vi "Calibration curve generator (for plot visualisation).vi"(0 "Calibration data":T1={"X cal.[]"=[0.18323830295620053, 0.5022759108677167, 0.5926494582411277, 0.6661572393359195, 0.7738522670991032, 0.8056162976693839, 0.8978854253288069, 0.9131465104685323, 0.998198602505461, 1.0026536354542668, 1.0697031684682123, 1.0921294784978217, 1.12634848007751], "Re cal.[]"=[0.05836901900647489, 0.22234941748039563, 0.3015014894413766, 0.37907259878050203, 0.5315212662031547, 0.5843186336351215, 0.7493379557739939, 0.7811312845686427, 0.9579100635301298, 0.968544779466997, 1.1278235480081842, 1.1845542549316277, 1.2707750850078616], "a1[]"=[0.5139845410306613, 0.694908421100499, 0.9655549133380104, 1.2354182702612118, 1.5388668488196042, 1.7253155968767342, 1.935875310920986, 2.080885331144939, 2.2328002605238204, 2.3813313947618693, 2.452594226248764, 2.5246632991683033], "a2[]"=[-0.567092642319511, 3.0111150428522957, -0.009461861177446703, 2.2004140825264833, 5.776179850523374, -0.22907956125341525, 19.477407826803766, -1.871103511573675, 70.58084557623488, -1.3220160025433672, 7.094218596447346, -0.2914365144530001], "a3[]"=[1.7775103256064757, -11.166529475918521, 16.733581628717324, -4.900141213800908, -59.63298736273686, 9.899216022714324, -643.3109334585097, 21.66651332028892, -8067.401298929666, 18.428518110921583, -163.1245085960374, 4.25840177969994]}, 5 "Overheat ratio":dbl=1.7, 7 "Gain":dbl=10.0, 9 "Offset (V)":dbl=0.512, 11 "N pts":i32=200, 12 "Vout_start (V)":dbl=0.0915928 format="%0.2f", 13 "Vout_end (V)":dbl=2.56055 format="%0.2f", 14 "Ta (°C)":dbl=20.43) -> ()   [LabVIEW 2022 SP3]
doc: "Generate spline interpolated calibration curve for plotting or testing purposes.\nPN 19-FEB-24."
uses:
  Ctls/Calibration data.ctl
  <vilib>/Analysis/1siggen.llb/Ramp Pattern by Samples.vi
  <vilib>/Analysis/NI_AALBase.lvlib
panel:
  out "U against Vout":cluster{dbl[], dbl[]}(graph)={[0.0915928, 0.10399962010050251, 0.11640644020100503, 0.12881326030150753, 0.14122008040201006, 0.15362690050251257, 0.16603372060301508, 0.1784405407035176, 0.1908473608040201, 0.20325418090452263, 0.21566100100502514, 0.22806782110552765, 0.24047464120603015, 0.25288146130653266, 0.2652882814070352, 0.27769510150753773, 0.2901019216080402, 0.3025087417085427, 0.31491556180904523, 0.32732238190954777, 0.3397292020100503, 0.3521360221105527, 0.36454284221105526, 0.3769496623115578, 0.38935648241206033, 0.40176330251256287, 0.4141701226130653, 0.42657694271356783, 0.43898376281407037, 0.4513905829145729, 0.46379740301507544, 0.47620422311557786, 0.4886110432160804, 0.5010178633165829, 0.5134246834170855, 0.525831503517588, 0.5382383236180904, 0.550645143718593, 0.5630519638190955, 0.575458783919598, 0.5878656040201006, 0.6002724241206031, 0.6126792442211055, 0.6250860643216081, 0.6374928844221106, 0.6498997045226131, 0.6623065246231157, 0.6747133447236181, 0.6871201648241206, 0.6995269849246232, 0.7119338050251257, 0.7243406251256282, 0.7367474452261307, 0.7491542653266332, 0.7615610854271357, 0.7739679055276383, 0.7863747256281408, 0.7987815457286432, 0.8111883658291458, 0.8235951859296483, 0.8360020060301508, 0.8484088261306534, 0.8608156462311558, 0.8732224663316583, 0.8856292864321609, 0.8980361065326634, 0.910442926633166, 0.9228497467336684, 0.9352565668341709, 0.9476633869346734, 0.960070207035176, 0.9724770271356785, 0.9848838472361809, 0.9972906673366835, 1.009697487437186, 1.0221043075376886, 1.034511127638191, 1.0469179477386934, 1.059324767839196, 1.0717315879396985, 1.084138408040201, 1.0965452281407035, 1.108952048241206, 1.1213588683417086, 1.133765688442211, 1.1461725085427135, 1.158579328643216, 1.1709861487437185, 1.183392968844221, 1.1957997889447236, 1.2082066090452261, 1.2206134291457287, 1.2330202492462312, 1.2454270693467338, 1.257833889447236, 1.2702407095477386, 1.2826475296482411, 1.2950543497487437, 1.3074611698492462, 1.3198679899497487, 1.3322748100502513, 1.3446816301507538, 1.3570884502512564, 1.3694952703517589, 1.3819020904522612, 1.3943089105527637, 1.4067157306532663, 1.4191225507537688, 1.4315293708542713, 1.4439361909547739, 1.4563430110552764, 1.468749831155779, 1.4811566512562815, 1.493563471356784, 1.5059702914572863, 1.5183771115577889, 1.5307839316582914, 1.543190751758794, 1.5555975718592965, 1.568004391959799, 1.5804112120603016, 1.592818032160804, 1.6052248522613066, 1.6176316723618092, 1.6300384924623115, 1.642445312562814, 1.6548521326633165, 1.667258952763819, 1.6796657728643216, 1.6920725929648242, 1.7044794130653267, 1.7168862331658292, 1.7292930532663318, 1.741699873366834, 1.7541066934673366, 1.7665135135678391, 1.7789203336683417, 1.7913271537688442, 1.8037339738693468, 1.8161407939698493, 1.8285476140703518, 1.8409544341708544, 1.853361254271357, 1.8657680743718592, 1.8781748944723617, 1.8905817145728643, 1.9029885346733668, 1.9153953547738694, 1.9278021748743719, 1.9402089949748744, 1.952615815075377, 1.9650226351758795, 1.977429455276382, 1.9898362753768843, 2.002243095477387, 2.0146499155778894, 2.027056735678392, 2.0394635557788945, 2.051870375879397, 2.0642771959798996, 2.076684016080402, 2.0890908361809046, 2.101497656281407, 2.1139044763819097, 2.1263112964824122, 2.1387181165829148, 2.1511249366834173, 2.16353175678392, 2.175938576884422, 2.1883453969849245, 2.200752217085427, 2.2131590371859295, 2.225565857286432, 2.2379726773869346, 2.250379497487437, 2.2627863175879397, 2.2751931376884422, 2.2875999577889448, 2.3000067778894473, 2.31241359798995, 2.3248204180904524, 2.337227238190955, 2.3496340582914574, 2.36204087839196, 2.3744476984924625, 2.386854518592965, 2.3992613386934676, 2.41166815879397, 2.424074978894472, 2.4364817989949747, 2.4488886190954773, 2.46129543919598, 2.4737022592964824, 2.486109079396985, 2.4985158994974874, 2.51092271959799, 2.5233295396984925, 2.535736359798995, 2.5481431798994976, 2.56055], [0.29664751804418277, 0.30662613588645926, 0.31654643206997446, 0.326410913704555, 0.33622213051710564, 0.34598267511226766, 0.35569518323367777, 0.3653623340258576, 0.37498685029670975, 0.3845714987806357, 0.3941190904022734, 0.4036324805408431, 0.4131145692951197, 0.42256830174901305, 0.4319966682377733, 0.44140270461480446, 0.45078949251910433, 0.4601601596433133, 0.469517880002384, 0.47886587420286675, 0.4882074097128137, 0.49754580113229246, 0.506884410464529, 0.5162266473876569, 0.5255759695270887, 0.5349358827285008, 0.5443099413314361, 0.5537017484435279, 0.563114956215335, 0.5725532661157939, 0.5820204292082937, 0.5915202464273579, 0.601056568855954, 0.6106332980034134, 0.6202543860839679, 0.6299238362959066, 0.6396457031013462, 0.6494240925066215, 0.6592631623432866, 0.669167122549744, 0.6791402354534771, 0.6891868160539103, 0.6993112323058823, 0.7095179054037294, 0.7198113100660003, 0.7301959748207745, 0.7406764822916041, 0.751257469484071, 0.7619436280729562, 0.7727397046900392, 0.783650501212498, 0.7946808750519365, 0.8058357394440255, 0.8171200637387619, 0.8285388736913374, 0.8400972517536395, 0.851800337366355, 0.8636533272516931, 0.8756614757067325, 0.8878300948973789, 0.9001645551529364, 0.9126702852613082, 0.9253527727647999, 0.9382175642565488, 0.951270265677565, 0.9645165426143937, 0.9779621205973903, 0.9916127853996161, 1.0054743833363466, 1.019552821565202, 1.0338540683868855, 1.0483841535465526, 1.0631491685357821, 1.0781552668951755, 1.0934086645175634, 1.1089156399518418, 1.1246825347074079, 1.1407986611009877, 1.1575328221098105, 1.1748799394868443, 1.1928113927677422, 1.2112981820539175, 1.230310926076732, 1.2498198602578183, 1.2697948347655108, 1.2902053125674107, 1.3110203674790741, 1.3322086822088324, 1.3537385463987164, 1.375577854661532, 1.3976941046140456, 1.4200543949062958, 1.4426254232470346, 1.4653734844252817, 1.4882644683280244, 1.5112638579540276, 1.5343367406199633, 1.557467407146475, 1.5806986219000898, 1.6040845345022898, 1.6276799191990272, 1.6515401778719652, 1.6757213430555151, 1.7002800809596976, 1.7252736944987899, 1.750760126325811, 1.776797961872767, 1.8034464323967587, 1.830765418031851, 1.8588154508467676, 1.8876577179084086, 1.9173540643511295, 1.9478784918610277, 1.9789923032726748, 2.010664694486561, 2.042881212325239, 2.0756272147037818, 2.1088878697208324, 2.142648154747884, 2.176892855516893, 2.2116065652061687, 2.2467736835245855, 2.2823784157940805, 2.3184047720304553, 2.354836566022473, 2.3916574144092664, 2.42885073575601, 2.46639974962797, 2.504287475662747, 2.5424967326409114, 2.5810101375548857, 2.6198101046761333, 2.6588788446206886, 2.6981983634129074, 2.738281785945614, 2.779718662870659, 2.822284966511532, 2.8657491971179, 2.909877303451982, 2.9544326712711304, 2.999170977667597, 3.043961837194833, 3.0888384286260444, 3.1338414473495217, 3.179012023287881, 3.224391722830543, 3.2700225507697382, 3.31594695223991, 3.3622078146605223, 3.408848469682385, 3.4559126951373083, 3.5034447169912846, 3.5514892113010568, 3.6000913061741238, 3.649296583732225, 3.699151082078164, 3.749701297266194, 3.8009941852757385, 3.8545121959120574, 3.9111270062211054, 3.96801918154515, 4.023791674126451, 4.079218171351564, 4.1343970977652855, 4.189426041787559, 4.244403612107474, 4.2994294420709425, 4.3546041940758435, 4.410029563974716, 4.4658082854849654, 4.522044134606581, 4.578841934047395, 4.636307557655805, 4.694547934861116, 4.75367105512128, 4.813785972378253, 4.875097432573927, 4.9413781580275264, 5.007061505535032, 5.072571495733658, 5.137998364566019, 5.203433264377012, 5.268968267748047, 5.334696371337724, 5.400711499728856, 5.467108509281911, 5.533983191994828, 5.601432279369256, 5.669553446283168, 5.73845078090282, 5.808877681951244, 5.880722772520939, 5.953131395834653, 6.02524268981699, 6.0970014894079885, 6.168808491811643, 6.240686283694641, 6.312657674972447, 6.384745699718895, 6.45697361707733]}
  out "Calibration curve":cluster{dbl[], dbl[]}(graph)={[0.18322804724684855, 0.18706364186223268, 0.1909083567135276, 0.194762191800734, 0.19862514712385096, 0.20249722268287929, 0.20637841847781838, 0.21026873450866887, 0.21416817077543057, 0.21807672727810296, 0.2219944040166866, 0.22592120099118104, 0.22985711820158672, 0.2338021556479034, 0.23775631333013145, 0.2417195912482703, 0.24569198940232026, 0.24967350779228126, 0.25366414641815327, 0.25766390527993627, 0.2616727843776309, 0.2656907837112362, 0.2697179032807525, 0.27375414308617974, 0.2777995031275183, 0.2818539834047682, 0.2859175839179287, 0.2899903046670003, 0.2940721456519831, 0.2981631068728767, 0.3022631883296819, 0.3063723900223979, 0.31049071195102484, 0.3146181541155628, 0.3187547165160119, 0.3229003991523721, 0.3270552020246433, 0.331219125132826, 0.3353921684769193, 0.3395743320569239, 0.3437656158728393, 0.34796601992466575, 0.3521755442124038, 0.3563941887360525, 0.3606219534956122, 0.36485883849108297, 0.3691048437224649, 0.37335996918975833, 0.3776242148929622, 0.38189758083207737, 0.38618006700710356, 0.39047167341804073, 0.39477240006488906, 0.3990822469476489, 0.40340121406631924, 0.40772930142090064, 0.41206650901139336, 0.4164128368377969, 0.42076828490011153, 0.42513285319833766, 0.4295065417324744, 0.4338893505025223, 0.4382812795084813, 0.44268232875035146, 0.4470924982281327, 0.45151178794182495, 0.4559401978914282, 0.4603777280769425, 0.4648243784983678, 0.46928014915570454, 0.47374504004895185, 0.4782190511781104, 0.48270218254318004, 0.48719443414416086, 0.4916958059810525, 0.4962062980538556, 0.5007259103625695, 0.5052546429071944, 0.5097924956877306, 0.5143394687041775, 0.5188955619565357, 0.5234607754448054, 0.5280351091689856, 0.5326185631290768, 0.5372111373250793, 0.5418128317569928, 0.5464236464248171, 0.5510435813285531, 0.5556726364682, 0.5603108118437578, 0.5649581074552266, 0.5696145233026064, 0.5742800593858978, 0.5789547157050998, 0.5836384922602127, 0.5883313890512368, 0.593033406078172, 0.5977445433410182, 0.6024648008397758, 0.6071941785744444, 0.6119326765450238, 0.6166802947515144, 0.621437033193916, 0.6262028918722289, 0.6309778707864522, 0.6357619699365875, 0.6405551893226332, 0.6453575289445903, 0.6501689888024585, 0.6549895688962372, 0.6598192692259277, 0.6646580897915288, 0.6695060305930413, 0.674363091630465, 0.6792292729037988, 0.6841045744130448, 0.6889889961582013, 0.6938825381392689, 0.6987852003562475, 0.7036969828091374, 0.7086178854979384, 0.7135479084226503, 0.7184870515832731, 0.7234353149798071, 0.7283926986122521, 0.7333592024806088, 0.7383348265848755, 0.743319570925054, 0.7483134355011433, 0.7533164203131438, 0.7583285253610557, 0.7633497506448776, 0.7683800961646117, 0.7734195619202564, 0.778468147911812, 0.7835258541392787, 0.7885926806026566, 0.793668627301946, 0.7987536942371459, 0.8038478814082569, 0.8089511888152789, 0.8140636164582122, 0.8191851643370569, 0.8243158324518117, 0.8294556208024785, 0.834604529389056, 0.8397625582115443, 0.8449297072699444, 0.8501059765642546, 0.8552913660944766, 0.8604858758606094, 0.8656895058626534, 0.8709022561006085, 0.8761241265744739, 0.8813551172842518, 0.8865952282299397, 0.8918444594115389, 0.8971028108290491, 0.9023702824824701, 0.907646874371803, 0.9129325864970463, 0.918227418858201, 0.9235313714552663, 0.9288444442882431, 0.9341666373571313, 0.93949795066193, 0.9448383842026398, 0.9501879379792606, 0.9555466119917925, 0.9609144062402356, 0.9662913207245898, 0.9716773554448556, 0.9770725104010315, 0.9824767855931189, 0.9878901810211171, 0.9933126966850265, 0.9987443325848477, 1.004185088720579, 1.0096349650922216, 1.0150939616997752, 1.0205620785432399, 1.0260393156226162, 1.0315256729379032, 1.0370211504891012, 1.04252574827621, 1.0480394662992303, 1.0535623045581617, 1.059094263053004, 1.0646353417837573, 1.0701855407504217, 1.075744859952997, 1.0813132993914836, 1.086890859065881, 1.0924775389761903, 1.0980733391224093, 1.1036782595045407, 1.1092923001225823, 1.1149154609765353, 1.1205477420663996, 1.1261891433921747], [0.058363747670762196, 0.06032698517798735, 0.0622787482235412, 0.06421953006732449, 0.06614983235391082, 0.06807016516382973, 0.06998104706496798, 0.07188300516409477, 0.07377657515850644, 0.07566230138779345, 0.07754073688572925, 0.07941244343227889, 0.0812779916057308, 0.08313796083494833, 0.084992939451744, 0.08684352474337384, 0.08869032300515443, 0.09053394959320019, 0.09237502897728259, 0.09421419479381055, 0.09605208989893259, 0.0978893664217589, 0.09972668581770713, 0.1015647189219676, 0.10340414600309086, 0.10524565681669587, 0.10708995065929988, 0.10893773642227048, 0.11078973264589766, 0.11264666757358782, 0.11450927920617972, 0.11637831535638019, 0.11825453370332326, 0.1201387018472492, 0.12203159736430534, 0.1239340078614683, 0.1258467310315874, 0.12777057470854997, 0.12970635692256668, 0.13165490595558052, 0.13361706039679452, 0.1355936691983228, 0.13758559173096255, 0.13959369784008557, 0.14161886790165454, 0.14366199287835782, 0.14572397437586668, 0.14780572469921416, 0.1499081669092938, 0.15203223487948256, 0.15417887335238215, 0.15634903799668326, 0.1585436954641511, 0.1607638234467319, 0.16301041073378025, 0.16528445726940977, 0.16758697420996319, 0.1699189839816038, 0.17228152033803, 0.1746756284183096, 0.1771023648048355, 0.1795627975814042, 0.18205800639141398, 0.1845890824961855, 0.18715712883340285, 0.18976326007567726, 0.19240860268923082, 0.19509429499270256, 0.19782148721607523, 0.2005913415597241, 0.20340503225358555, 0.20626374561645008, 0.20916868011537304, 0.21212104642520957, 0.21512206748826884, 0.21817297857409207, 0.22127502733934842, 0.22444578548513175, 0.2277381385007244, 0.2311510872692946, 0.2346790008738187, 0.23831617374569886, 0.24205682528390277, 0.2458950994733428, 0.2498250645024897, 0.25384071238022576, 0.25793595855193463, 0.26210464151483104, 0.2663405224325235, 0.27063728474881943, 0.2749885338007659, 0.2793877964309272, 0.28382852059890185, 0.28830407499207406, 0.2928077486356074, 0.29733275050167274, 0.3018722117141923, 0.3064230415795843, 0.3109936537488839, 0.31559470185865446, 0.32023696243684624, 0.32493133549524156, 0.3296888451230401, 0.33452064008158955, 0.33943799440025557, 0.3444523079734398, 0.34957510715873075, 0.3548180453762093, 0.36019290370888624, 0.3657115915042871, 0.37138614697718214, 0.37722873781344984, 0.38323424898956837, 0.38935571816712133, 0.39558708481102367, 0.40192550533907667, 0.4083680990025867, 0.4149119477075346, 0.4215540958353958, 0.4282915500636342, 0.4351212791858553, 0.4420402139316307, 0.4490452467859839, 0.4561332318085439, 0.46330098445236223, 0.47054528138239793, 0.47786286029366193, 0.48525041972904076, 0.492704618896766, 0.5002220774875664, 0.5077993754914767, 0.5154330530143106, 0.5231196100938108, 0.5308555065154456, 0.538741696745195, 0.5468941715916474, 0.5552688548566628, 0.5638202002531749, 0.5725021595031672, 0.581268180071684, 0.5900701927868274, 0.5988825450378743, 0.6077117645637394, 0.6165658579555083, 0.6254529172964759, 0.6343811205423512, 0.6433587319021552, 0.6523941022197882, 0.6614956693562654, 0.6706719585726465, 0.6799315829136191, 0.6892832435917761, 0.6987357303725596, 0.708297921959882, 0.7179787863824291, 0.7277873813806229, 0.7377328547942839, 0.7478244449509487, 0.7583538155966658, 0.769492464337402, 0.7806856831006844, 0.7916586105178613, 0.8025634652749435, 0.8134196118531676, 0.8242462502308603, 0.8350627811186233, 0.8458888068225827, 0.8567441321091113, 0.8676487650710315, 0.8786229179953013, 0.8896870082321736, 0.9008616590658423, 0.912167700586556, 0.9236261705642302, 0.9352583153235144, 0.9470855906203608, 0.9591482790789689, 0.9721886428120401, 0.9851114757599565, 0.9980002016224707, 1.0108725738189281, 1.0237465260657208, 1.0366401731306525, 1.049571811588569, 1.062559920578239, 1.0756231625604982, 1.0887803840776444, 1.102050616514101, 1.1154530768583313, 1.1290082438775628, 1.14286434457621, 1.1569994661677827, 1.1712454596894255, 1.1854329553204201, 1.1995510996423357, 1.2136787275992855, 1.2278202829921947, 1.2419802535449431, 1.2561631710833219, 1.270373611714295]}
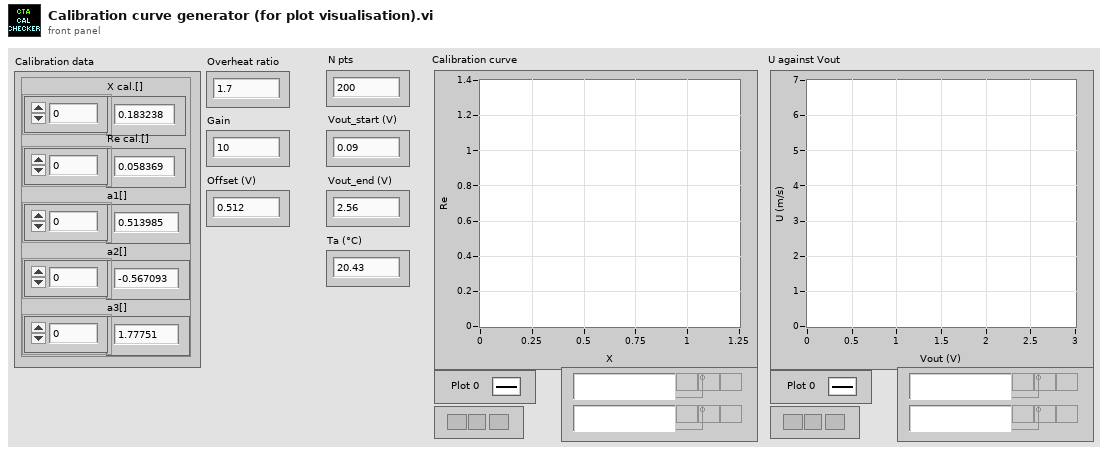
[diagram p1: front panel]
types:
  T1 = typedef "Calibration data.ctl" = cluster{"X cal.[]":dbl[], "Re cal.[]":dbl[], "a1[]":dbl[], "a2[]":dbl[], "a3[]":dbl[]}
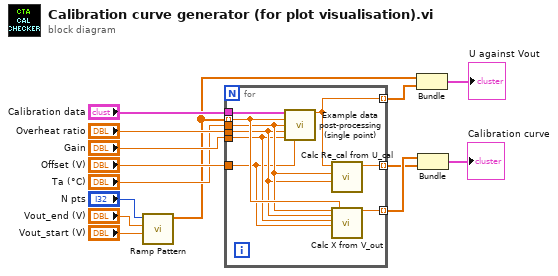
[diagram p0: block diagram]
diagram:
  n1 = call-poly <vilib>:"Ramp Pattern.vi"("start"="Vout_start (V)", "end"="Vout_end (V)", "samples"="N pts") -> ("Ramp Pattern"=w3:dbl[])  [unwired: 7 in, 1 out]
  n2 = for {
    tunnel: "Offset (V)" -> [w15]
    tunnel: "Gain" -> [w16]
    tunnel: "Overheat ratio" -> [w17]
    tunnel: "Calibration data" -> [w23]
    tunnel: w3 -> [w19] mode=indexing
    tunnel: "Ta (°C)" -> [w18]
    tunnel: [w22] -> w5 mode=indexing
    tunnel: [w21] -> w6 mode=indexing
    tunnel: [w20] -> w2 mode=indexing
    n3 = call "Example data post-processing (single point).vi"("Calibration data"=w23, "V_out (V)"=w19, "Ta (°C)"=w18, "Overheat ratio (Rw / R0)"=w17, "Gain"=w16, "Offset (V)"=w15) -> ("U (m/s)"=w20:dbl)  [unwired: 9 in]
    n4 = call "Calc Re_cal from U_cal.vi"("Overheat ratio (Rw / R0)"=w17, "Ta (°C)"=w18, "U_cal (m/s)"=w20) -> ("Re"=w22:dbl)  [unwired: 8 in]
    n5 = call "Calc X from V_out.vi"("Ta (°C)"=w18, "Overheat ratio (Rw / R0)"=w17, "Gain"=w16, "Offset (V)"=w15, "V_out (V)"=w19) -> ("X"=w21:dbl)  [unwired: 14 in]
  }
  n6 = Bundle("Ramp Pattern"=w3, w2) -> (→"U against Vout":cluster{"Ramp Pattern":dbl[], dbl[]})  [unwired: 1 in]
  n7 = Bundle(w6, w5) -> (→"Calibration curve":cluster{dbl[], dbl[]})  [unwired: 1 in]
